vi "VCS Set Velocity Profile.vi"(8 "error in (no error)":errorcluster, 10 "velocity profile":T1, 11 "axis in":cluster{"keyHandle":u32, "nodeId":u16}={"keyHandle"=0, "nodeId"=1}) -> (0 "error out":errorcluster, 3 "axis out":cluster{"keyHandle":u32, "nodeId":u16}={"keyHandle"=0, "nodeId"=1})   [LabVIEW 2019]
doc: "<B>VCS Set Velocity Profile</B> writes all velocity profile parameters."
uses:
  Resources/EposCmd.dll
  Resources/EposCmd64.dll
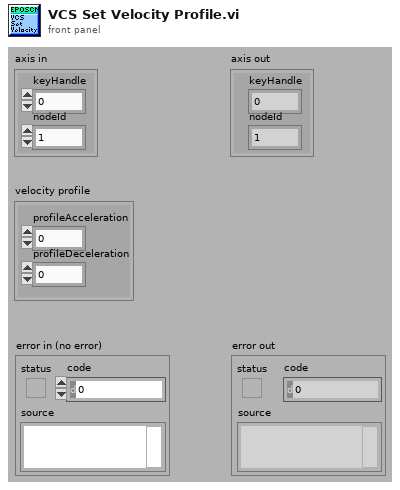
[diagram p1: front panel]
types:
  T1 = cluster{"profileAcceleration":u32, "profileDeceleration":u32}
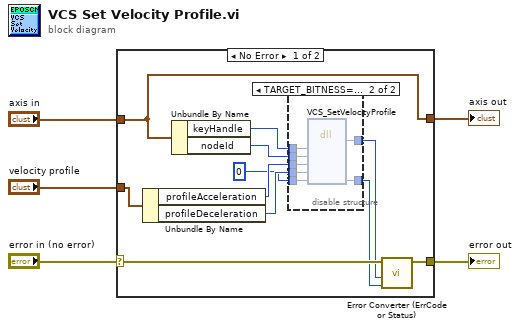
[diagram p0: block diagram]
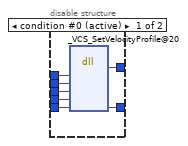
[diagram p2: hidden frame]
diagram:
  n1 = case shown="No Error" "error in (no error)" {
    selector: "error in (no error)" -> [w16 w32]
    tunnel: [w15 w32] -> w4
    tunnel: "axis in" -> [w7 w31]
    tunnel: "velocity profile" -> [w11 _]
    tunnel: [w7 w31] -> w1
    frame No Error {
      n2 = Unbundle By Name(w11) -> ("profileAcceleration"=w10:u32, "profileDeceleration"=w9:u32)
      n3 = Unbundle By Name(w7) -> ("keyHandle"=w13:u32, "nodeId"=w12:u16)
      n4 = disable-structure shown="TARGET_BITNESS==64" {
        disable-tunnel: [w23 w30] -> w14
        disable-tunnel: w13 -> [w22 w29]
        disable-tunnel: w12 -> [w21 w28]
        disable-tunnel: w10 -> [w20 w27]
        disable-tunnel: w9 -> [w19 w26]
        disable-tunnel: u32 0 ("pErrorCode") -> [w18 w25]
        disable-tunnel: [w17 w24] -> w6
        frame condition #0 (active) {
          n5 = dll-call lib="C:/Projeto em LabVIEW/EPOS-LabVIEW-Instrument-Driver-En/LabVIEW/maxon EPOS/Resources/EposCmd.*" fn="_VCS_SetVelocityProfile@20"("KeyHandle"=w22, "NodeId"=w21, "ProfileAcceleration"=w20, "ProfileDeceleration"=w19, "pErrorCode"=w18) -> (w17:i32, "pErrorCode"=w23:u32)  [unwired: 7 in, 2 out]
        }
        frame condition #1 {
          n6 = dll-call lib="C:/setup/Resources/EposCmd64.*" fn="VCS_SetVelocityProfile" ("EposCmd.dll:_VCS_SetVelocityProfile@20")("KeyHandle"=w29, "NodeId"=w28, "ProfileAcceleration"=w27, "ProfileDeceleration"=w26, "pErrorCode"=w25) -> ("Rückgabetyp"=w24:i32, "pErrorCode"=w30:u32)  [unwired: 7 in, 2 out]
        }
      }
      n7 = call "Error Converter (ErrCode or Status).vi"("error code"=w14, "return type"=w6, "error in (no error)"=w16) -> ("error out"=w15:errorcluster)  [unwired: 7 in]
    }
    frame Error {
    }
  }
  "error out" <- w4
  "axis out" <- w1
